vi "Current Time.vi"(8 "error in (no error)":errorcluster, 11 "Model in":refnum<class "Model.lvclass">) -> (0 "error out":errorcluster, 2 "Time":dbl, 3 "Model out":refnum<class "Model.lvclass">)   [LabVIEW 2016, in "Model.lvclass"]
uses:
  Model.lvclass
  Model.lvclass/Model.ctl
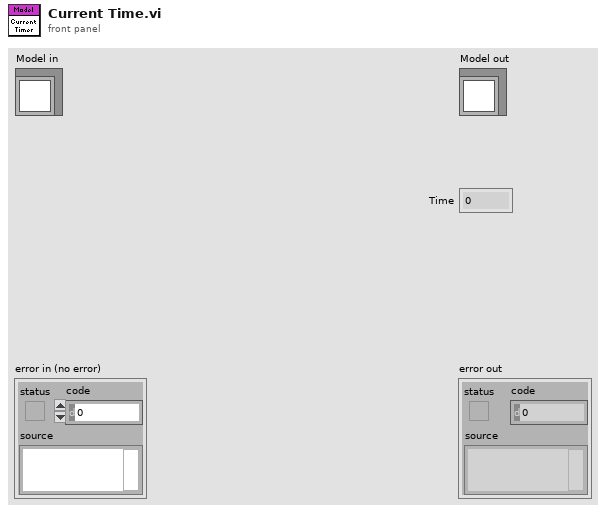
[diagram p1: front panel]
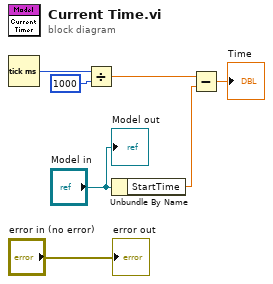
[diagram p0: block diagram]
diagram:
  n1 = Tick Count (ms)() -> (millisecond timer value=w3:u32)
  n2 = Divide(x=w3, y=u32 1000) -> (x/y=w1:dbl)
  n3 = Unbundle By Name("Model in") -> ("StartTime"=w7:dbl)
  n4 = Subtract(x=w1, y=w7) -> (x-y=→"Time":dbl)
  "error out" <- "error in (no error)"
  "Model out" <- "Model in"
